vi "PH_Trendviewer_Powermeter.ProcEvents.vi"(0 "i ref in":refnum<vi>, 5 "error in (no error)":errorcluster) -> (14 "i ref out":refnum<vi>, 19 "error out":errorcluster)   [LabVIEW 2014, in "PH_Trendviewer_Powermeter.lvlib"]
doc: "This method is used to define the events the object will listen to. Add your own events here."
uses:
  PH_Trendviewer_Powermeter.lvlib
  CSCore/BaseProcess/BaseProcess.event definition.ctl
  CSCore/CAEObj/CAEObj.event definition.ctl
  CSCore/BaseProcess/BaseProcess.descriptor string definition.ctl
  CSCore/BaseProcess/BaseProcess.lvlib
  CSCore/CAEObj/CAEObj.lvlib
  PH_Common/PH_Common.lvlib
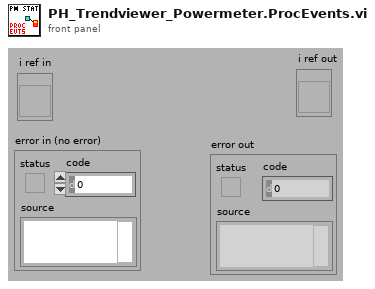
[diagram p1: front panel]
types:
  T1 = typedef "BaseProcess.lvlib/BaseProcess.event definition.ctl" = cluster{"CAEEvtDef":T2, "Data Descriptor":T3}
  T2 = typedef "CAEObj.lvlib/CAEObj.event definition.ctl" = cluster{"URL":string, "enable":bool, "ignoreResID":bool}
  T3 = typedef "BaseProcess.lvlib/BaseProcess.descriptor string definition.ctl" = string
  T4 = typedef "PH_Trendviewer_Powermeter.lvlib/PH_Trendviewer_Powermeter.i attribute.ctl" = cluster{"GUI Refs ":cluster{"Status":refnum<vi>, "Result Graph":refnum<vi>, "Mean Data":refnum<vi>, "Std Dev Data":refnum<vi>, "Dummy Mean":refnum<vi>, "Dummy Std Dev":refnum<vi>, "Export Data":refnum<vi>, "Stat or Trend":refnum<vi>, "Delete":refnum<vi>, "Powermeter":refnum<vi>, "Start":refnum<vi>}, "Powermeter":string, "Stat or Trend":bool, "Start":bool, "Data":cluster{"Time Stamp":timestamp, "Energy [J]":dbl}[], "Datasets strored":i32, "Dataarray Size":i32}
  T5 = typedef "PH_Common.lvlib/PH_DIM.Event Declarer.ctl" = cluster{"Service Name":string, "Selector":string}
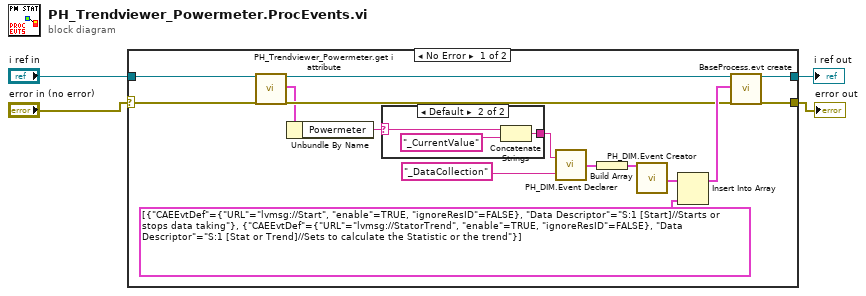
[diagram p0: block diagram]
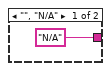
[diagram p2: hidden frame]
diagram:
  n1 = case shown="No Error" "error in (no error)" {
    selector: "error in (no error)" -> [w13 w25]
    tunnel: "i ref in" -> [w11 w24]
    tunnel: [w19 w24] -> w3
    tunnel: [w18 w25] -> w2
    frame No Error {
      n2 = call "PH_Trendviewer_Powermeter.get i attribute.vi"("i ref in"=w11, "error in (no error)"=w13) -> ("i ref out"=w10:refnum<vi>, "i attribute"=w9:T4, "error out"=w12:errorcluster)  [unwired: 15 in]
      n3 = Unbundle By Name(w9) -> ("Powermeter"=w8:string)
      n4 = case shown="Default" w8 {
        selector: w8 -> [_ w23]
        tunnel: ["N/A" w22] -> w7
        frame "", "N/A" {
        }
        frame Default {
          n5 = Concatenate Strings(w23, "_CurrentValue") -> (w22:string)
        }
      }
      n6 = call "PH_DIM.Event Declarer.vi"("Selector"="_DataCollection", "Service Name"=w7) -> ("declared DIM Event"=w16:T5)
      n7 = Build Array(w16) -> (w5:T5[])
      n8 = call "PH_DIM.Event Creator.vi"("Trendnotifier Services"=w5) -> ("DIM Service Events"=w17:T1[])  [unwired: 18 in]
      n9 = Insert Into Array(array=w17, new element=T1[] [{"CAEEvtDef"={"URL"="lvmsg://Start", "enable"=TRUE, "ignoreResID"=FALSE}, "Data Descriptor"="S:1 [Start]//Starts or stops data taking"}, {"CAEEvtDef"={"URL"="lvmsg://StatorTrend", "enable"=TRUE, "ignoreResID"=FALSE}, "Data Descriptor"="S:1 [Stat or Trend]//Sets to calculate the Statistic or the trend"}] ("new events")) -> (w15:T1[])  [unwired: 1 in]
      n10 = call "BaseProcess.evt create.vi"("i ref in"=w10, "newEvents"=w15, "error in (no error)"=w12) -> ("i ref out"=w19:refnum<vi>, "error out"=w18:errorcluster)  [unwired: 13 in, 2 out]
    }
    frame Error {
    }
  }
  "i ref out" <- w3
  "error out" <- w2
